vi "Tool-Kalman Filter (with noise).vi"(3 "프런트패널 윈도우:모니터":u16) -> ()   [LabVIEW 2015]
uses:
  SUB_Load and Save Controls.llb/RWC_Actions.ctl
  <vilib>/ptbypt/NI_PtbyPt.lvlib
panel:
  in  "Export to Excel":bool
  in  "Interval time (ms)":u32=1 min=1 max=5000
  in  "Noise Lavel":dbl=1.48e-05 format="%.8f"
  out "Graph":waveform(dbl)[](graph)=[{"t0"=timestamp(3554674983.6106663 s since 1904-01-01), "dt"=11.49265718460083, "Y"=[0.9971512413550824]}, {"t0"=timestamp(3554674983.6106663 s since 1904-01-01), "dt"=11.49265718460083, "Y"=[0.9971599783084714]}]
  in  "x input":dbl(slide)=0.99715 step=1.0 scale=0.99715..0.99735 scale format="%#_6f"
  in  "Exit":bool
  out "Ready":bool=TRUE
  out "Numeric Control":i32=766
  in  "R":dbl=0.65 min=0.0 max=1000.0 step=0.1 format="%#.3f"
  in  "Q":dbl=0.004 min=0.0 max=1000.0 step=0.01 format="%#.5f"
  out "Kalman X":dbl=0.9971512413550824 format="%.5f"
  out "Real X":dbl=0.9971599783084714 format="%.5f"
  # "CDC Filter Simulation"
  # "Filter Gain setting"
  # "Q: 예측 노이즈 공분산\n    값이 작을수록 무겁게 동작\nR: 측정 노이즈 공분산\n    값이 클수록 무겁게 동작"
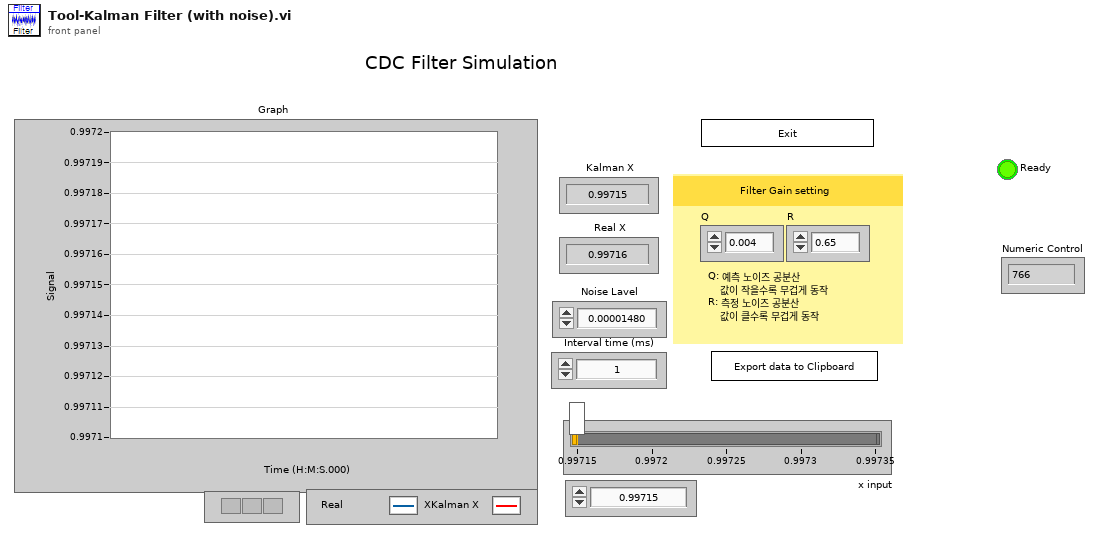
[diagram p1: front panel]
types:
  T1 = typedef "RWC_Actions.ctl" = enum16{"Read", "Write", "Read and Create"}
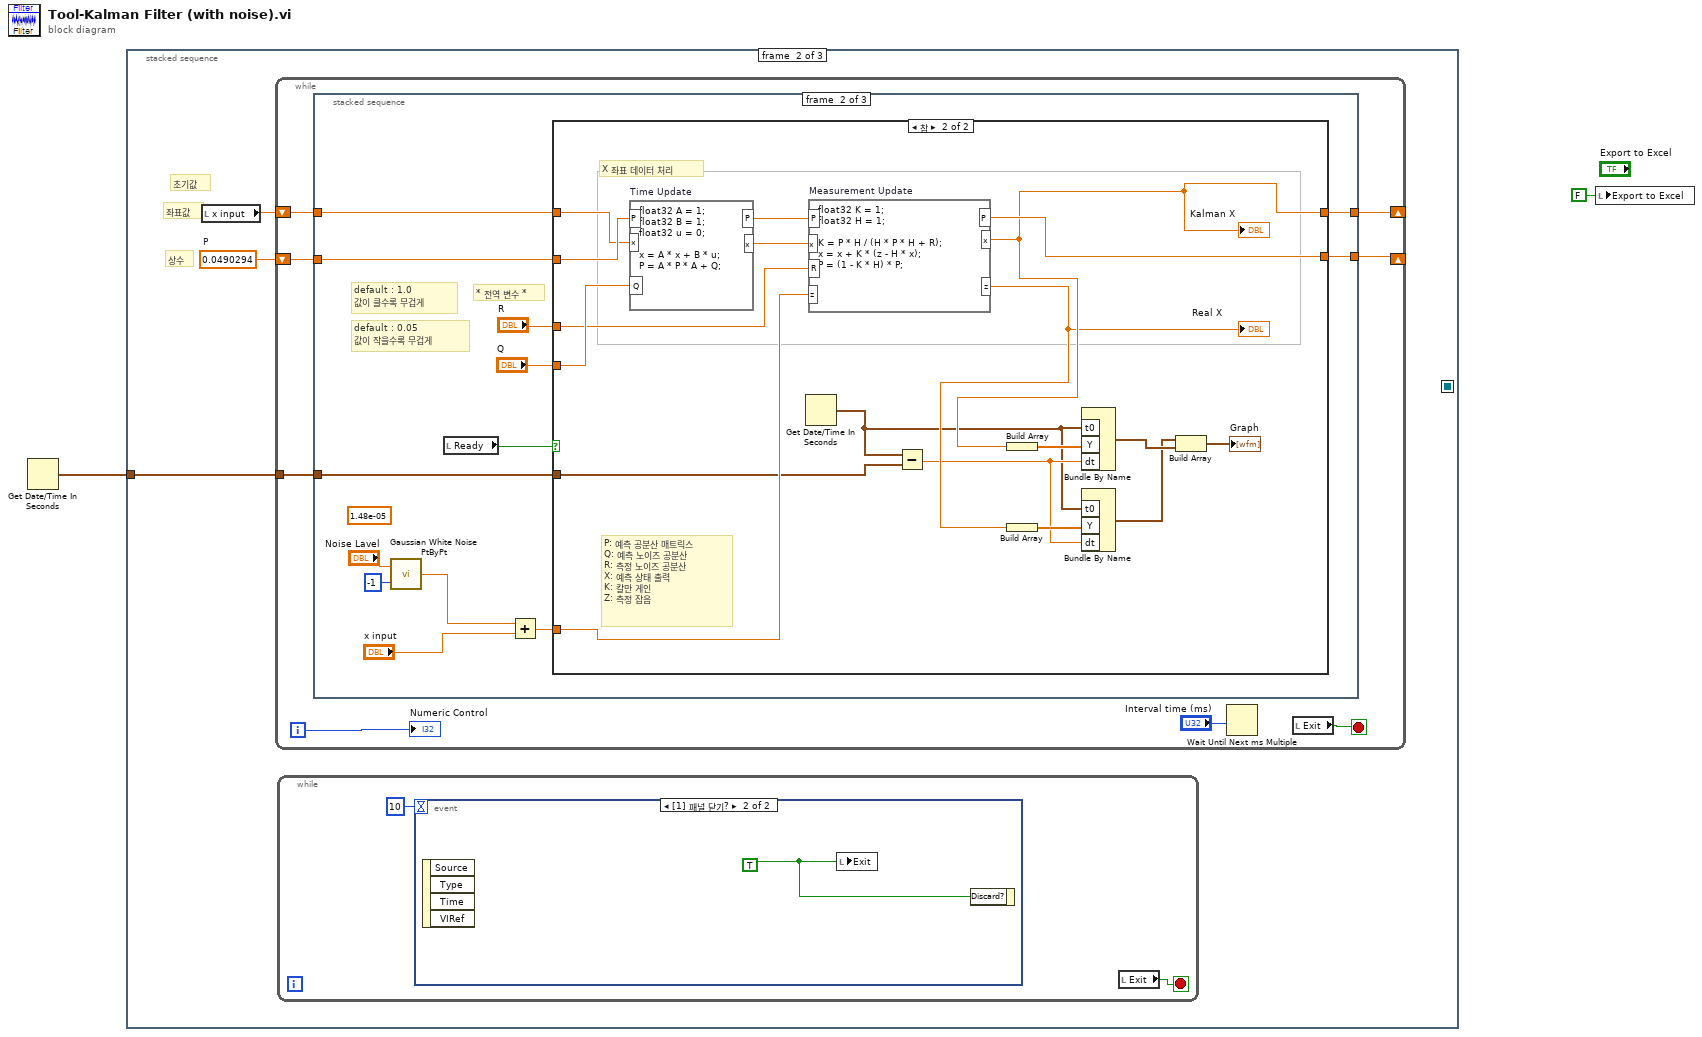
[diagram p0: block diagram]
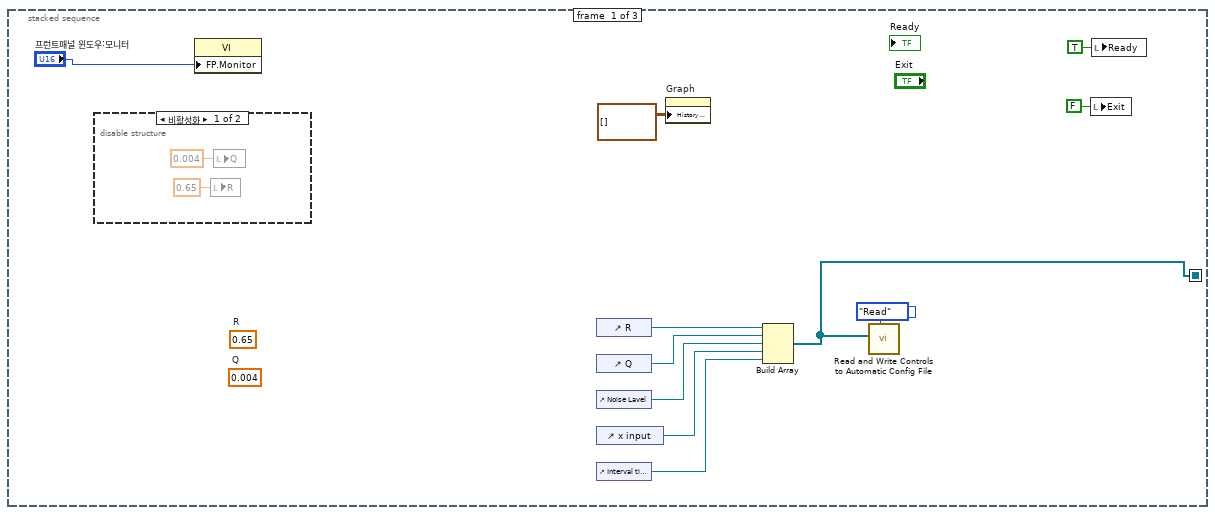
[diagram p2: hidden frame]
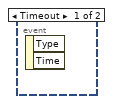
[diagram p4: hidden frame]
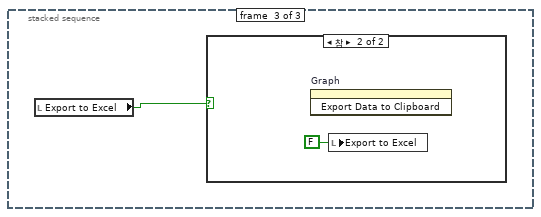
[diagram p7: hidden frame]
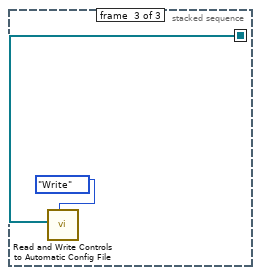
[diagram p9: hidden frame]
diagram:
  n1 = Get Date/Time In Seconds() -> (seconds since 1Jan1904=w2:timestamp)
  n2 = stacked-sequence {
    seq-local: [w8 _ _] -> [_ _ w65]
    tunnel: w2 -> [_ w17 _]
    frame #0 {
      (unwired) 0.004  # Q
      (unwired) 0.65  # R
      n3 = disable-structure shown="비활성화" {
        frame Disabled {
          n4 = local write "R"(0.65 ("R")) -> ()
          n5 = local write "Q"(0.004 ("Q")) -> ()
        }
        frame Enabled {
        }
      }
      n6 = property class="VI"("FP.Monitor"="프런트패널 윈도우:모니터") -> ()  [unwired: 2 in, 2 out]
      n7 = control-ref of="R"() -> (w7:refnum<vi>)
      n8 = control-ref of="Q"() -> (w6:refnum<vi>)
      n9 = control-ref of="Noise Lavel"() -> (w5:refnum<vi>)
      n10 = control-ref of="x input"() -> (w4:refnum<vi>)
      n11 = control-ref of="Interval time (ms)"() -> (w3:refnum<vi>)
      n12 = property on="Graph" class="WFChart (엄격한)"("History Data"=waveform(dbl)[][] [] ("히스토리 데이터")) -> ()  [unwired: 2 in, 2 out]
      n13 = Build Array(w7, w6, w5, w4, w3) -> (w8:refnum<vi>[])
      n14 = call "Read and Write Controls to Automatic Config File.vi"("Action"=RWC_Actions."Read", "Control References"=w8) -> ()  [unwired: 9 in, 1 out]
      n15 = local write "Exit"(FALSE ("Exit")) -> ()
      n16 = local write "Ready"(TRUE ("Ready")) -> ()
    }
    frame #1 {
      w18 = 0.0490294  # P
      # "좌표값"
      # "상수"
      # "초기값"
      n17 = local read "x input"() -> (w16:dbl)
      n18 = while {
        shift-right: [w26] -> _
        shift-left: w16 -> [w28]
        shift-right: [w27] -> _
        shift-left: w18 -> [w29]
        tunnel: w17 -> [w24]
        i -> [w23]
        stop <- w25 stop-if-true
        n19 = stacked-sequence {
          tunnel: w29 -> [_ w37 _]
          tunnel: w28 -> [_ w42 _]
          tunnel: [_ w41 _] -> w27
          tunnel: [_ w40 _] -> w26
          tunnel: w24 -> [_ w31 _]
          frame #0 {
          }
          frame #1 {
            (unwired) 1.48e-05 ("standard deviation")
            # "* 전역 변수 *"
            # "default : 0.05\n값이 작을수록 무겁게"
            # "default : 1.0\n값이 클수록 무겁게"
            n20 = call <vilib>:"Gaussian White Noise PtByPt.vi"("seed"=-1, "standard deviation"="Noise Lavel") -> ("Gaussian white noise"=w35:dbl)  [unwired: 1 in]
            n21 = local read "Ready"() -> (w36:bool)
            n22 = Add(x=w35, y="x input") -> (x+y=w32:dbl)
            n23 = case shown="참" w36 {
              tunnel: w37 -> [w43 w62]
              tunnel: w42 -> [w44 w59]
              tunnel: [w43 w58] -> w41
              tunnel: [w44 w53] -> w40
              tunnel: "Q" -> [_ w57]
              tunnel: "R" -> [_ w56]
              tunnel: w32 -> [_ w55]
              tunnel: w31 -> [_ w46]
              frame False {
              }
              frame True {
                # "P: 예측 공분산 매트릭스\nQ: 예측 노이즈 공분산\nR: 측정 노이즈 공분산\nX: 예측 상태 출력 \nK: 칼만 게인\nZ: 측정 잡음"
                # "X 좌표 데이터 처리"
                n24 = formula code="float32 A = 1;\nfloat32 B = 1;\nfloat32 u = 0;\n\nx = A * x + B * u;\nP = A * P * A + Q;" "Time Update"("x"=w59, "P"=w62, "Q"=w57) -> ("x"=w61:dbl, "P"=w60:dbl)
                n25 = Get Date/Time In Seconds() -> (seconds since 1Jan1904=w45:timestamp)
                n26 = formula code="float32 K = 1;\nfloat32 H = 1;\n\nK = P * H / (H * P * H + R);\nx = x + K * (z - H * x);\nP = (1 - K * H) * P;" "Measurement Update"("x"=w61, "P"=w60, "z"=w55, "R"=w56) -> ("x"=w53:dbl, "P"=w58:dbl, "z"=w50:dbl)
                "Kalman X" <- w53
                "Real X" <- w50
                n27 = Subtract(x=w45, y=w46) -> (x-y=w49:dbl)
                n28 = Build Array(w53) -> (w54:dbl[])
                n29 = Build Array(w50) -> (w52:dbl[])
                n30 = Bundle By Name("t0"=w45, "Y"=w54, "dt"=w49) -> (w51:waveform(dbl))  [unwired: 1 in]
                n31 = Bundle By Name("t0"=w45, "Y"=w52, "dt"=w49) -> (w48:waveform(dbl))  [unwired: 1 in]
                n32 = Build Array(w48, w51) -> (→"Graph":waveform(dbl)[])
              }
            }
          }
          frame #2 {
            n33 = local read "Export to Excel"() -> (w63:bool)
            n34 = case shown="참" w63 {
              frame False {
              }
              frame True {
                n35 = invoke on="Graph" class="WFChart (엄격한)" method="Export Data to Clipboard"() -> ()  [unwired: 3 in, 3 out]
                n36 = local write "Export to Excel"(FALSE ("Export to Excel")) -> ()
              }
            }
          }
        }
        n37 = Wait Until Next ms Multiple(millisecond multiple="Interval time (ms)") -> ()  [unwired: 1 out]
        n38 = local read "Exit"() -> (w25:bool)
        "Numeric Control" <- w23
      }
      n39 = while {
        stop <- w19 stop-if-true
        n40 = event shown="[1] 패널 닫기?" {
          selector: _ -> [_ _]
          dyn-events: _ -> [_ _]
          timeout: 10 -> [_ _]
          event Timeout {
            n41 = event-data() -> ()  [unwired: 1 in, 2 out]
          }
          event Panel Close? {
            w21 = TRUE ("Exit")
            n42 = event-data() -> ()  [unwired: 1 in, 4 out]
            n43 = local write "Exit"(w21) -> ()
            n44 = event-data("Discard?"=w21) -> ()  [unwired: 1 in, 1 out]
          }
        }
        n45 = local read "Exit"() -> (w19:bool)
      }
    }
    frame #2 {
      n46 = call "Read and Write Controls to Automatic Config File.vi"("Action"=RWC_Actions."Write", "Control References"=w65) -> ()  [unwired: 9 in, 1 out]
    }
  }
  n47 = local write "Export to Excel"(FALSE ("Export to Excel")) -> ()
